vi "Threshold 1D T-Periodic Array (xN).vi"(7 "Period":dbl, 9 "Search Values":dbl[](array[numeric]), 11 "X":dbl[](array[numeric])) -> (3 "Interpolated Indices":dbl[](array[numeric]))   [LabVIEW 2021, in "Arrays.lvlib"]
uses:
  Arrays.lvlib
  9126c8e0-c887-40cd-9668-65afecc2b031.vi
  Comparison/Comparison.lvlib
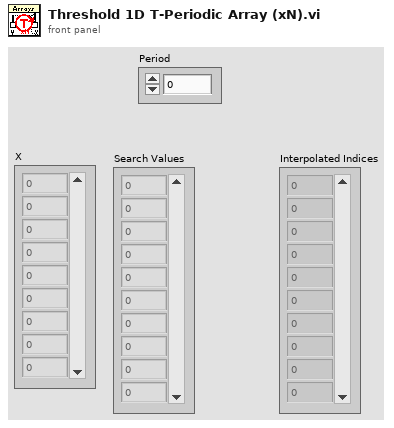
[diagram p1: front panel]
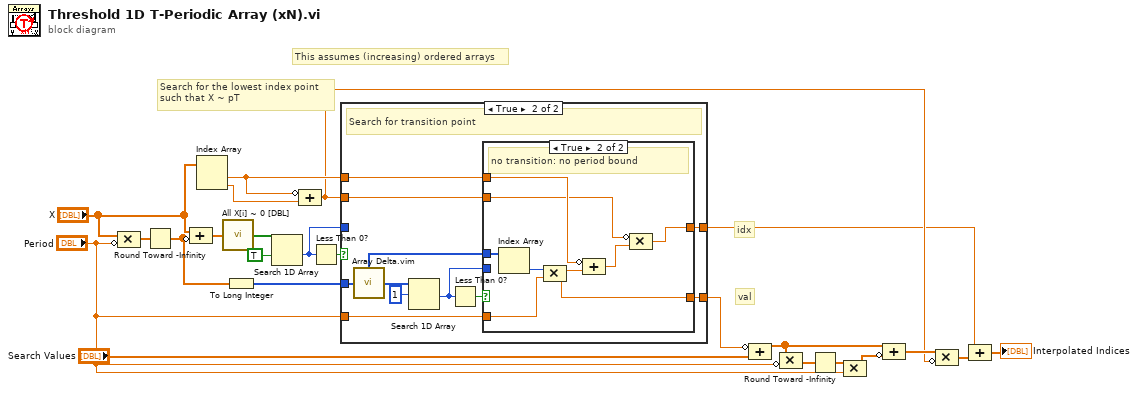
[diagram p0: block diagram]
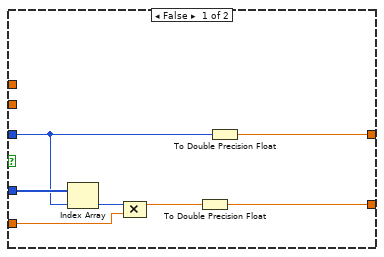
[diagram p2: hidden frame]
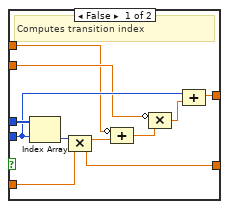
[diagram p3: hidden frame]
diagram:
  # "val"
  # "idx"
  # "Search for the lowest index point\nsuch that X ~ pT"
  # "This assumes (increasing) ordered arrays"
  n1 = Compound Arithmetic op=MULTIPLY("X", invert "Period") -> (w23:dbl[])
  n2 = Round Toward -Infinity(1:w23) -> (0:w18:dbl[])
  n3 = Compound Arithmetic op=ADD("X", invert w18) -> (w22:dbl[])
  n4 = Index Array(array="X") -> (element #1=w5:dbl, element #2=w6:dbl)  [unwired: 2 in]
  n5 = call "All X[i] ~ 0 [DBL].vi"("X Array"=w22) -> ("~ 0 ?"=w21:bool[])  [unwired: 14 in]
  n6 = To Long Integer(number=w18) -> (32bit integer=w16:i32[])
  n7 = Search 1D Array(1D array=w21, element=TRUE) -> (index of element=w17:i32)  [unwired: 1 in]
  n8 = Compound Arithmetic op=ADD(invert w5, w6) -> (w4:dbl)
  n9 = Less Than 0?(x=w17) -> (x < 0?=w19:bool)
  n10 = case shown="True" w19 {
    tunnel: w16 -> [w29 w36]
    tunnel: w17 -> [w28 _]
    tunnel: [w30 w34] -> w3
    tunnel: "Period" -> [w24 w35]
    tunnel: [w26 w33] -> w15
    tunnel: w4 -> [_ w32]
    tunnel: w5 -> [_ w31]
    frame False {
      n11 = Index Array(array=w29, index=w28) -> (element=w27:i32)
      n12 = Compound Arithmetic op=MULTIPLY(w27, w24) -> (w25:dbl)
      n13 = To Double Precision Float(number=w25) -> (double precision float=w26:dbl)
      n14 = To Double Precision Float(number=w28) -> (double precision float=w30:dbl)
    }
    frame True {
      # "Search for transition point"
      n15 = call "Array Delta.vim"("A"=w36) -> ("A[i+1]-A[i]"=w40:i32[])  [unwired: 8 in]
      n16 = Search 1D Array(1D array=w40, element=1) -> (index of element=w37:i32)  [unwired: 1 in]
      n17 = Less Than 0?(x=w37) -> (x < 0?=w38:bool)
      n18 = case shown="True" w38 {
        tunnel: w37 -> [w45 _]
        tunnel: w36 -> [w50 w58]
        tunnel: w35 -> [w48 w56]
        tunnel: [w44 w54] -> w34
        tunnel: [w43 w53] -> w33
        tunnel: w32 -> [w42 w51]
        tunnel: w31 -> [w41 w52]
        frame False {
          # "Computes transition index"
          n19 = Index Array(array=w50, index=w45) -> (element=w49:i32)
          n20 = Compound Arithmetic op=MULTIPLY(w49, w48) -> (w43:dbl)
          n21 = Compound Arithmetic op=ADD(invert w41, w43) -> (w47:dbl)
          n22 = Compound Arithmetic op=MULTIPLY(invert w42, w47) -> (w46:dbl)
          n23 = Compound Arithmetic op=ADD(w45, w46) -> (w44:dbl)
        }
        frame True {
          # "no transition: no period bound"
          n24 = Index Array(array=w58) -> (element=w57:i32)  [unwired: 1 in]
          n25 = Compound Arithmetic op=MULTIPLY(w57, w56) -> (w53:dbl)
          n26 = Compound Arithmetic op=ADD(invert w52, w53) -> (w55:dbl)
          n27 = Compound Arithmetic op=MULTIPLY(invert w51, w55) -> (w54:dbl)
        }
      }
    }
  }
  n28 = Compound Arithmetic op=ADD(invert w15, "Search Values") -> (w10:dbl[])
  n29 = Compound Arithmetic op=MULTIPLY(w10, invert "Period") -> (w14:dbl[])
  n30 = Round Toward -Infinity(1:w14) -> (0:w13:dbl[])
  n31 = Compound Arithmetic op=MULTIPLY(w13, "Period") -> (w9:dbl[])
  n32 = Compound Arithmetic op=ADD(w10, invert w9) -> (w8:dbl[])
  n33 = Compound Arithmetic op=MULTIPLY(w8, invert w4) -> (w2:dbl[])
  n34 = Compound Arithmetic op=ADD(w3, w2) -> (→"Interpolated Indices":dbl[])
